vi "WriteImageFileJpeg2000.vi"(4 "Advanced Options":T1={"Wavelet transform mode"=enum."integer", "Use multi-component transform?"=FALSE, "Max wavelet transform level"=5, "Quantization step size"=0.0}, 6 "Compression Ratio":sgl=50.0, 7 "Color Palette":T2[](array[typedef]), 8 "error in":errorcluster, 9 "Lossless":bool=TRUE, 10 "File Path":path, 11 "Image Reference In":T3) -> (0 "error out":errorcluster, 3 "Image Reference Out":T3)   [LabVIEW 2024, in "OpenLvVision_Image.lvlib" / "File.lvlib"]
doc: "Saves the image to a file in the chosen format."
uses:
  File.lvlib
  Management/TypeDef/Image.ctl
  TypeDef/ColorPaletteValue.ctl
  TypeDef/Jpeg2000AdvancedOptions.ctl
  Management/Management.lvlib
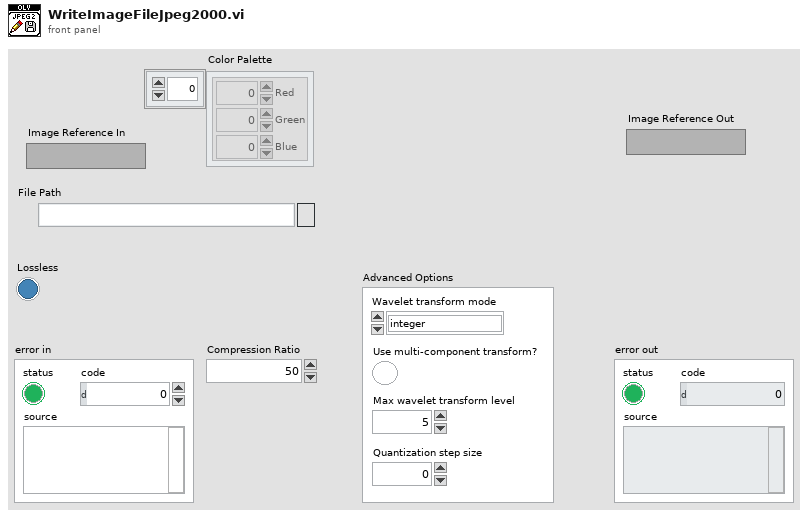
[diagram p1: front panel]
types:
  T1 = typedef "OpenLvVision_Image.lvlib/File.lvlib/Jpeg2000AdvancedOptions.ctl" = cluster{"Wavelet transform mode":enum16{"integer", "floating point"}, "Use multi-component transform?":bool, "Max wavelet transform level":i32, "Quantization step size":sgl}
  T2 = typedef "OpenLvVision_Image.lvlib/File.lvlib/ColorPaletteValue.ctl" = cluster{"Red":u8, "Green":u8, "Blue":u8}
  T3 = typedef "OpenLvVision_Image.lvlib/Management.lvlib/Image.ctl" = refnum<image>
  T4 = typedef "IMAQ Image.ctl" = refnum<image>
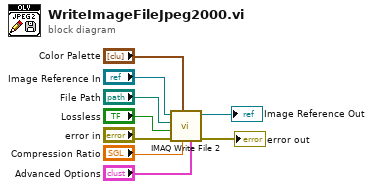
[diagram p0: block diagram]
diagram:
  n1 = call-poly "IMAQ Write File 2"("Advanced Options"="Advanced Options", "Compression Ratio"="Compression Ratio", "Color Palette"="Color Palette", "error in (no error)"="error in", "Lossless? (true)"="Lossless", "File Path"="File Path", "Image"="Image Reference In") -> ("error out"=→"error out":errorcluster, "Image Out (duplicate)"=→"Image Reference Out":T4)  [unwired: 3 in]
